vi "xboxOpen.vi"(0 "error in (no error)":errorcluster) -> (1 "xboxID":refnum<k1>, 2 "xboxError":errorcluster)   [LabVIEW 2017]
uses:
  globalDevices.vi
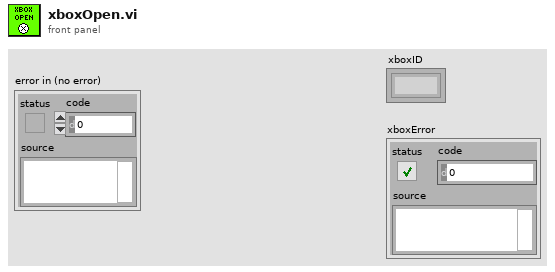
[diagram p1: front panel]
types:
  T1 = cluster{"axes total":u32, "buttons total":u32, "pov total":u32, "device name":string}[]
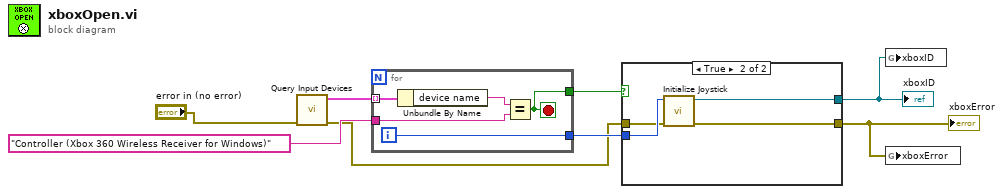
[diagram p0: block diagram]
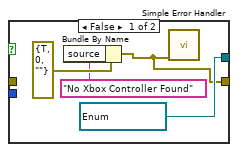
[diagram p2: hidden frame]
diagram:
  n1 = call <vilib>:"Query Input Devices.vi"("error in (no error)"="error in (no error)") -> ("error out"=w1:errorcluster, "joystick info"=w8:T1)  [unwired: 7 in, 2 out]
  n2 = for {
    tunnel: w8 -> [w13] mode=indexing
    tunnel: "Controller (Xbox 360 Wireless Receiver for Windows)" -> [w11]
    tunnel: [w10] -> w5
    tunnel: [w9] -> w6
    i -> [w10]
    stop <- w9 stop-if-true
    n3 = Unbundle By Name(w13) -> ("device name"=w12:string)
    n4 = Equal?(x=w12, y=w11) -> (x = y?=w9:bool)
  }
  n5 = case shown="True" w6 {
    tunnel: w5 -> [_ w21]
    tunnel: w1 -> [_ w20]
    tunnel: [w15 w19] -> w2
    tunnel: [w14 w18] -> w3
    frame False {
      w15 = refnum<k1> refnum items=["JOYSTICK"] ("device ID")
      n6 = Bundle By Name(cluster=errorcluster {"status"=TRUE, "code"=0, "source"=""} ("error constant"), "source"="No Xbox Controller Found") -> (w14:errorcluster)
      n7 = call <vilib>:"Simple Error Handler.vi"("error in (no error)"=w14) -> ()  [unwired: 4 in, 5 out]
    }
    frame True {
      n8 = call <vilib>:"Initialize Joystick.vi"("error in (no error)"=w20, "device index"=w21) -> ("error out"=w18:errorcluster, "device ID"=w19:refnum<k1>)  [unwired: 8 in]
    }
  }
  "xboxError" <- w3
  "xboxID" <- w2
  n9 = global write "globalDevices.vi" "xboxID"(w2) -> ()
  n10 = global write "globalDevices.vi" "xboxError"(w3) -> ()
